vi "Control_UI.vi"(7 "Disabled":T1, 8 "error in (no error)":errorcluster, 11 "Array":refnum<vi>[](array[refnum])) -> (0 "error out":errorcluster)   [LabVIEW 2026]
uses:
  controls/Control_Enum.ctl
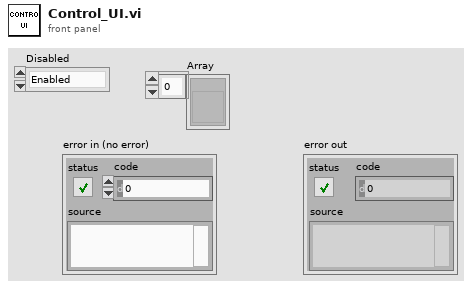
[diagram p1: front panel]
types:
  T1 = typedef "Control_Enum.ctl" = enum8{"Enabled", "Disabled", "Disabled and Grayed Out"}
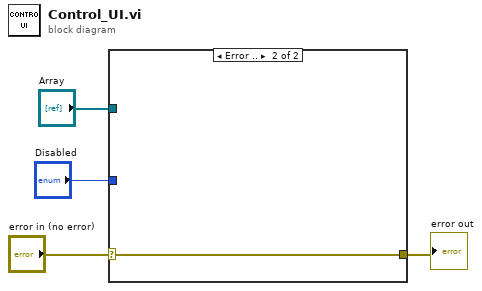
[diagram p0: block diagram]
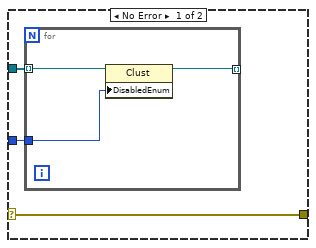
[diagram p2: hidden frame]
diagram:
  n1 = case shown="Error .." "error in (no error)" {
    selector: "error in (no error)" -> [w5 w11]
    tunnel: "Array" -> [w7 _]
    tunnel: "Disabled" -> [w6 _]
    tunnel: [w5 w11] -> w1
    frame No Error {
      n2 = for {
        tunnel: w7 -> [w10] mode=indexing
        tunnel: w6 -> [w9]
        tunnel: [w8] -> _ mode=indexing
        n3 = property class="Clust"(reference=w10, "DisabledEnum"=w9) -> (reference out=w8:refnum<vi>)  [unwired: 1 in, 1 out]
      }
    }
    frame Error {
    }
  }
  "error out" <- w1
